vi "Expected Info.vi"() -> (2 "Length Map":cluster{i32[]}[](array[cluster]), 3 "Expected Digit Info":T1[](array[typedef])=[{"Expected"=[0, 1, 2, 4, 5, 6], "Actual"=[]}, {"Expected"=[2, 5], "Actual"=[]}, {"Expected"=[0, 2, 3, 4, 6], "Actual"=[]}, {"Expected"=[0, 2, 3, 5, 6], "Actual"=[]}, {"Expected"=[1, 2, 3, 5], "Actual"=[]}, {"Expected"=[0, 1, 3, 5, 6], "Actual"=[]}, {"Expected"=[0, 1, 3, 4, 5, 6], "Actual"=[]}, {"Expected"=[0, 2, 5], "Actual"=[]}, {"Expected"=[0, 1, 2, 3, 4, 5, 6], "Actual"=[]}, {"Expected"=[0, 1, 2, 3, 5, 6], "Actual"=[]}], 5 "Empty Segment Map":cluster{i32[]}[](array[cluster]))   [LabVIEW 2020]
uses:
  Digit Info.ctl
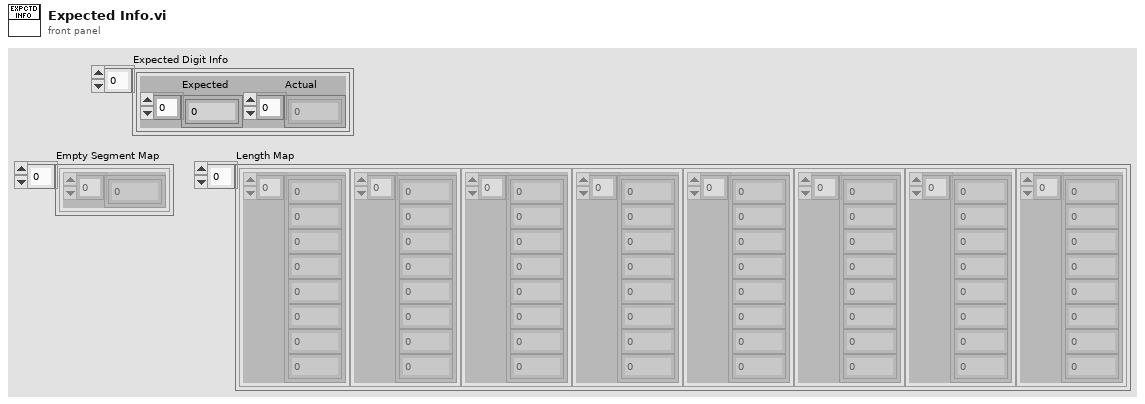
[diagram p1: front panel]
types:
  T1 = typedef "Digit Info.ctl" = cluster{"Expected":i32[], "Actual":i32[]}
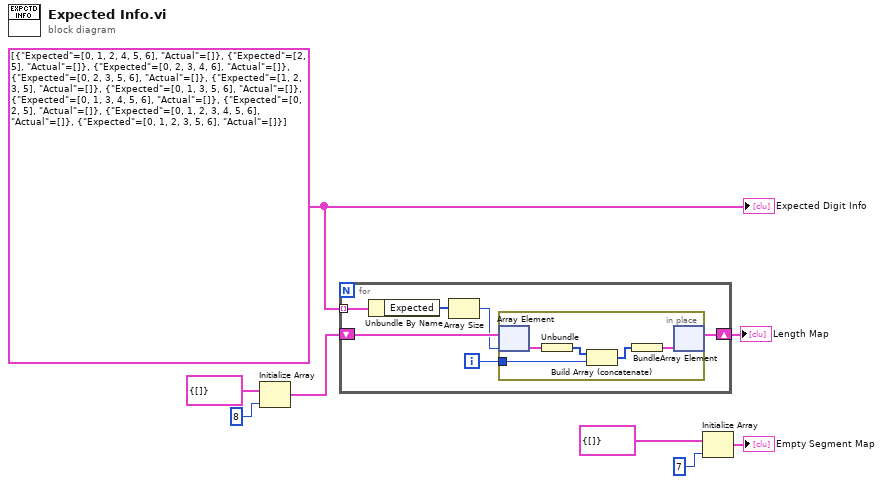
[diagram p0: block diagram]
diagram:
  w8 = T1[] [{"Expected"=[0, 1, 2, 4, 5, 6], "Actual"=[]}, {"Expected"=[2, 5], "Actual"=[]}, {"Expected"=[0, 2, 3, 4, 6], "Actual"=[]}, {"Expected"=[0, 2, 3, 5, 6], "Actual"=[]}, {"Expected"=[1, 2, 3, 5], "Actual"=[]}, {"Expected"=[0, 1, 3, 5, 6], "Actual"=[]}, {"Expected"=[0, 1, 3, 4, 5, 6], "Actual"=[]}, {"Expected"=[0, 2, 5], "Actual"=[]}, {"Expected"=[0, 1, 2, 3, 4, 5, 6], "Actual"=[]}, {"Expected"=[0, 1, 2, 3, 5, 6], "Actual"=[]}]
  n1 = Initialize Array(cluster{i32[]} {[]}, 8 ("dimension size")) -> (w2:cluster{i32[]}[])
  n2 = for {
    tunnel: w8 -> [w14] mode=indexing
    shift-right: [w9] -> w1
    shift-left: w2 -> [w11]
    i -> [w12]
    n3 = Unbundle By Name(w14) -> ("Expected"=w13:i32[])
    n4 = Array Size(array=w13) -> (size(s)=w10:i32)
    n5 = in-place {
      in-place-border: w12 -> [w19]
      n6 = in-place-array #1(w11, w10) -> (w18:cluster{i32[]})
      n7 = Unbundle(w18) -> (w17:i32[])
      n8 = Build Array (concatenate)(w17, w19) -> (w16:i32[])
      n9 = Bundle(w16) -> (w15:cluster{i32[]})  [unwired: 1 in]
      n10 = in-place-array #1(w15) -> (w9:cluster{i32[]}[])  [unwired: 1 out]
    }
  }
  "Length Map" <- w1
  n11 = Initialize Array(cluster{i32[]} {[]}, 7 ("dimension size")) -> (→"Empty Segment Map":cluster{i32[]}[])
  "Expected Digit Info" <- w8
